vi "Validate_Proper Indentation.vi"(0 "Functions in":T1[](array[typedef]), 11 "error in (no error)":errorcluster) -> (4 "Functions":T1[](array[typedef]), 6 "Validation message":T2[](array[typedef]), 15 "error out":errorcluster)   [LabVIEW 2016, in "scripts manager.lvclass"]
uses:
  scripts manager.lvclass
  common/Line Details.ctl
  common/Validate_message.ctl
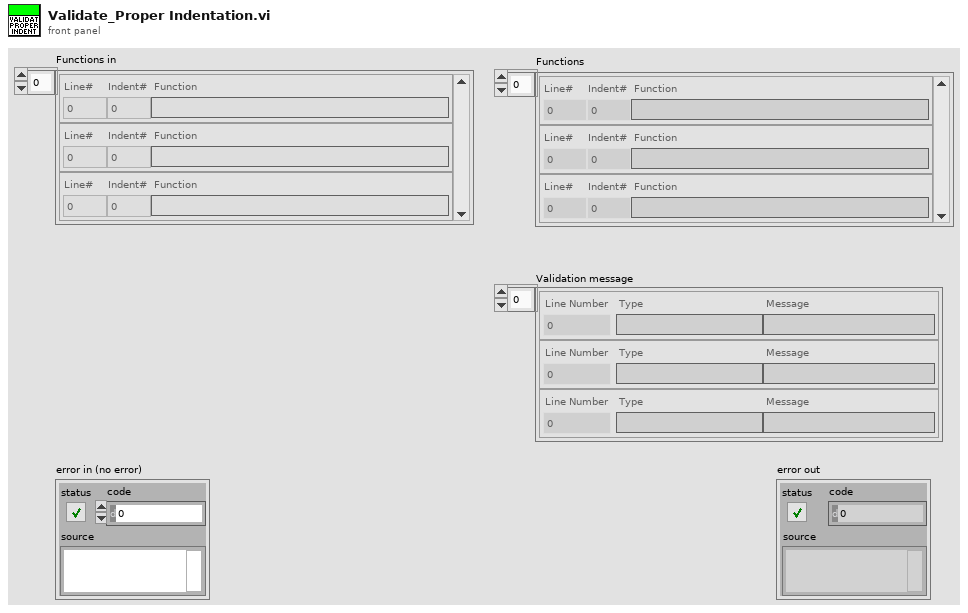
[diagram p1: front panel]
types:
  T1 = typedef "Line Details.ctl" = cluster{"Line#":i64, "Indent#":i64, "Function":string}
  T2 = typedef "Validate_message.ctl" = cluster{"Line Number":i64, "Type":string, "Message":string}
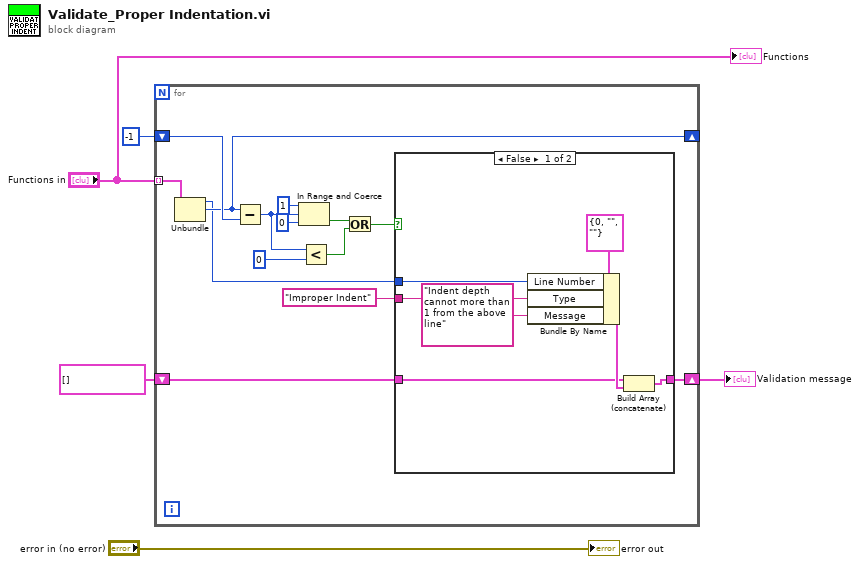
[diagram p0: block diagram]
diagram:
  n1 = for {
    tunnel: "Functions in" -> [w13] mode=indexing
    shift-right: [w11] -> _
    shift-left: i64 -1 ("Indent") -> [w19]
    shift-right: [w7] -> w1
    shift-left: T2[] [] -> [w6]
    n2 = Unbundle(w13) -> ("Line#"=w10:i64, "Indent#"=w11:i64)  [unwired: 1 out]
    n3 = Subtract(x=w11, y=w19) -> (x-y=w8:i64)
    n4 = In Range and Coerce(upper limit=i64 1, x=w8, lower limit=i64 0) -> (In Range?=w15:bool)  [unwired: 1 out]
    n5 = Less?(x=w8, y=i64 0) -> (x < y?=w14:bool)
    n6 = Or(x=w15, y=w14) -> (x .or. y?=w12:bool)
    n7 = case shown="False" w12 {
      tunnel: w10 -> [w25 _]
      tunnel: "Improper Indent" ("Type") -> [w24 _]
      tunnel: [w21 w27] -> w7
      tunnel: w6 -> [w20 w27]
      frame False {
        n8 = Bundle By Name(cluster=T2 {"Line Number"=0, "Type"="", "Message"=""} ("Message"), "Line Number"=w25, "Type"=w24, "Message"="Indent depth cannot more than 1 from the above line") -> (w22:T2)
        n9 = Build Array (concatenate)(w20, w22) -> (w21:T2[])
      }
      frame True {
      }
    }
  }
  "Validation message" <- w1
  "error out" <- "error in (no error)"
  "Functions" <- "Functions in"
